vi "ParseSolverString.vi"(9 "Moves Enum":T1, 11 "String":string) -> (3 "Array":u16[](array[numeric]))   [LabVIEW 2017]
uses:
  Controls/RubikMoves.ctl
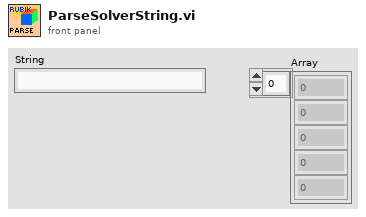
[diagram p1: front panel]
types:
  T1 = typedef "RubikMoves.ctl" = enum16{"U", "U'", "F", "F'", "D", "D'", "B", "B'", "L", "L'", "R", "R'"}
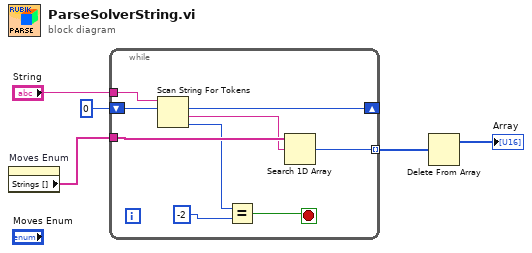
[diagram p0: block diagram]
diagram:
  n1 = property on="Moves Enum" class="Enum (strict)"() -> ("Strings []"=w1:string[])  [unwired: 2 in, 2 out]
  n2 = while {
    tunnel: "String" -> [w14]
    shift-right: [w7] -> _
    shift-left: 0 ("offset past token") -> [w13]
    tunnel: [w6] -> w2 mode=indexing
    tunnel: w1 -> [w12]
    stop <- w10 stop-if-true
    n3 = Scan String For Tokens(8:w13, 9:w14) -> (0:w8:i32, 1:w11:string, 2:w7:i32)  [unwired: 4 in, 1 out]
    n4 = Equal?(x=w8, y=-2) -> (x = y?=w10:bool)
    n5 = Search 1D Array(1D array=w12, element=w11) -> (index of element=w6:i32)  [unwired: 1 in]
  }
  n6 = Delete From Array(array=w2) -> (array with subset deleted=→"Array":i32[])  [unwired: 2 in, 1 out]
